vi "Joystick Simulator.vi"(3 "Degrees":dbl) -> (0 "Y":dbl, 1 "X":dbl)   [LabVIEW 2015]
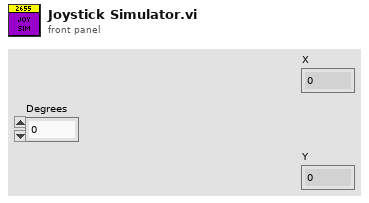
[diagram p1: front panel]
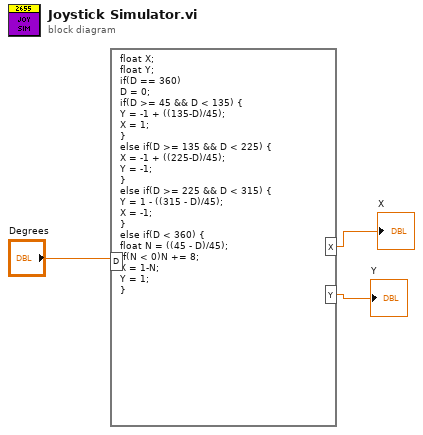
[diagram p0: block diagram]
diagram:
  n1 = formula code="float X;\nfloat Y;\nif(D == 360)\nD = 0;\nif(D >= 45 && D < 135) {\nY = -1 + ((135-D)/45);\nX = 1;\n}\nelse if(D >= 135 && D < 225) {\nX = -1 + ((225-D)/45);\nY = -1;\n}\nelse if(D >= 225 && D < 315) {\nY = 1 - ((315 - D)/45);\nX = -1;\n}\nelse if(D < 360) {\nfloat N = ((45 - D)/45);\nif(N < 0)N += 8;\nX = 1-N;\nY = 1;\n}"("D"="Degrees") -> ("X"=→"X":dbl, "Y"=→"Y":dbl)
